vi "TcA01-011_CloneObject.vi"(1 "Input buffer":T3="1", 3 "Invocation info":T2, 5 "error in (no error)":errorcluster, 6 "Add log to result?":bool) -> (16 "Test Data":T1 {"Numeric Measurement" format="%.2f"}, 19 "error out":errorcluster)   [LabVIEW 2009]
doc: "Test case template."
uses:
  Shared/Support_InputBuffer.ctl
  Shared/Support_InvocationInfo.ctl
  Shared/Support_TestData.ctl
  TestClasses/G#SubClass1_class/G#SubClass1.lvclass
  <vilib>/addons/_AddQ/G#Object/G#Object.lvclass
panel:
  in  "Test name":string="TcA01-011 Clone object"
  out "Test result":bool
  out "Result":string
  # "Verify that clone object works."
  # "Sub test case"
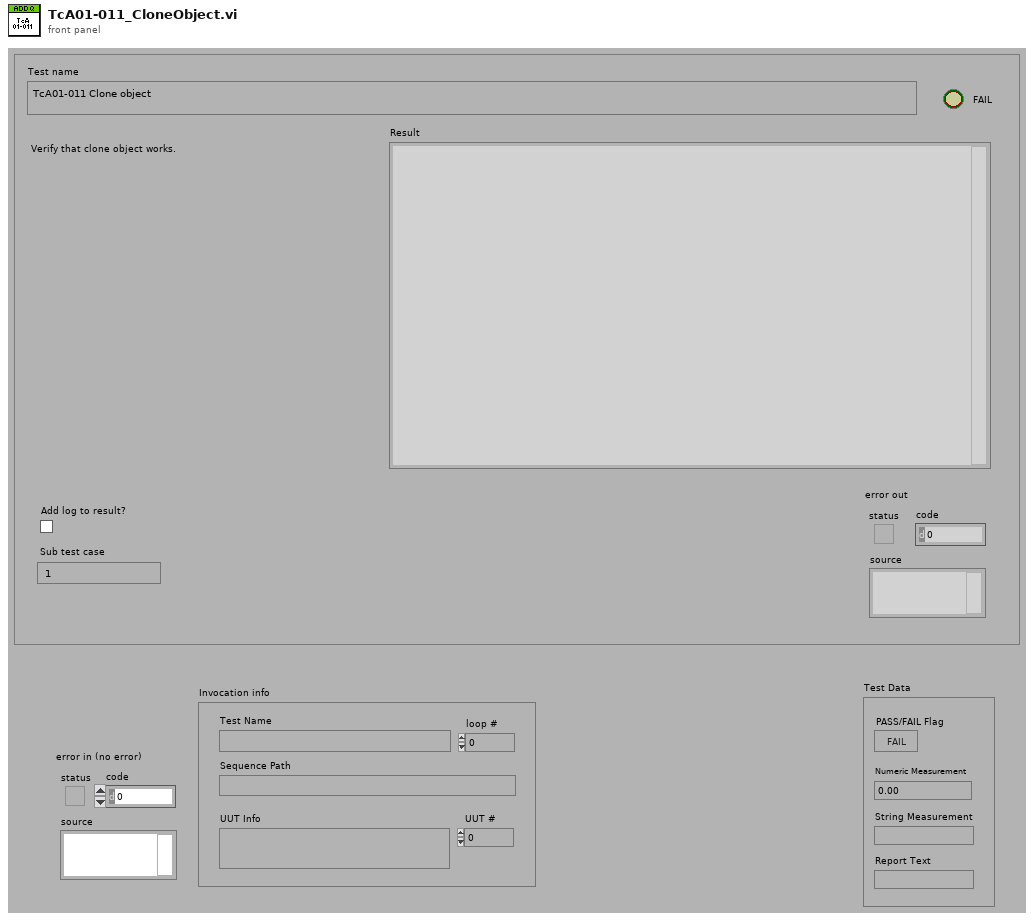
[diagram p1: front panel]
types:
  T1 = typedef "Support_TestData.ctl" = cluster{"PASS/FAIL Flag":bool, "Numeric Measurement":dbl, "String Measurement":string, "Report Text":string}
  T2 = typedef "Support_InvocationInfo.ctl" = cluster{"UUT #":i32, "loop #":i32, "UUT Info":string, "Test Name":string, "Sequence Path":path}
  T3 = typedef "Support_InputBuffer.ctl" = string
  T4 = typedef "Support_ResultType.ctl" = cluster{"Pass":bool, "Comment":string, "MeasurementValue":dbl}
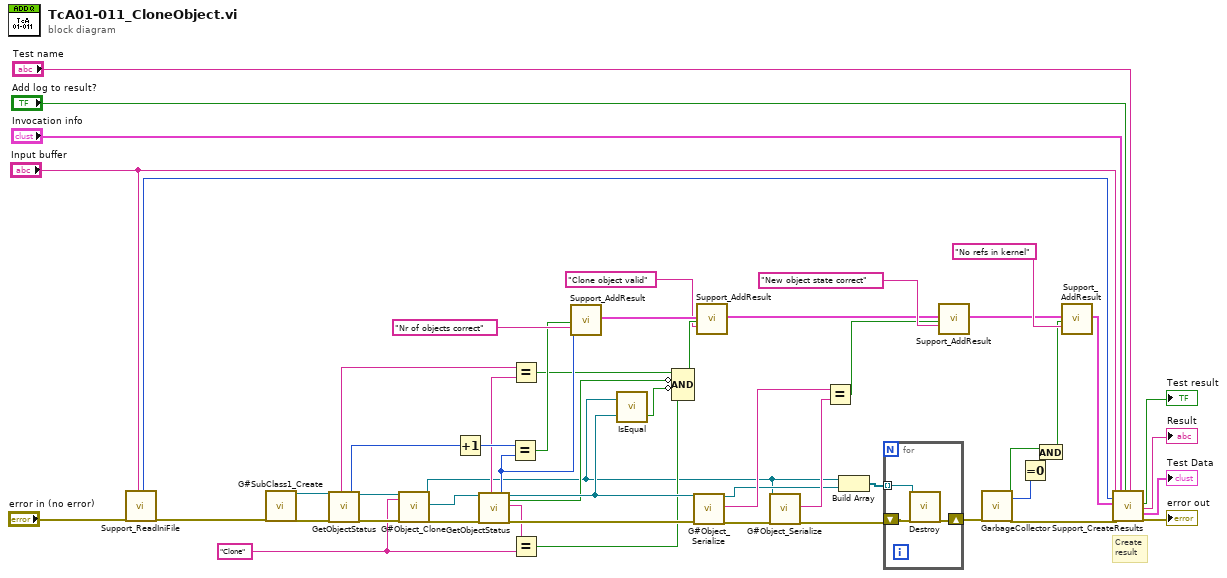
[diagram p0: block diagram]
diagram:
  w1 = "Clone" ("new object name")
  # "Create\nresult"
  n1 = call "Support_ReadIniFile.vi"("error in (no error)"="error in (no error)", "Sub test case"="Input buffer") -> ("Timer start"=w43:u32, "error out"=w34:errorcluster)  [unwired: 10 in, 6 out]
  n2 = call "G#SubClass1_Create.vi"("error in (no error)"=w34) -> ("reference out"=w32:refnum<class "G#SubClass1.lvclass">, "error out"=w33:errorcluster)  [unwired: 16 in, 1 out]
  n3 = call-dynamic "GetObjectStatus.vi"("reference in"=w32, "error in (no error)"=w33) -> ("full class name"=w10:string, "# of objects"=w27:i32, "reference out"=w30:refnum<class "G#SubClass1.lvclass">, "error out"=w31:errorcluster)  [unwired: 6 in, 8 out]
  n4 = call <vilib>:"G#Object_Clone.vi"("reference in"=w30, "new object name"=w1, "error in (no error)"=w31) -> ("reference out"=w3:refnum<class "G#SubClass1.lvclass">, "new object reference out"=w29:refnum<class "G#SubClass1.lvclass">, "error out"=w28:errorcluster)  [unwired: 14 in]
  n5 = Increment(x=w27) -> (x+1=w26:i32)
  n6 = call-dynamic "GetObjectStatus.vi"("reference in"=w29, "error in (no error)"=w28) -> ("full class name"=w11:string, "# of objects"=w25:i32, "reference out"=w19:refnum<class "G#SubClass1.lvclass">, "not a refnum?"=w16:bool, "object name"=w8:string, "error out"=w23:errorcluster)  [unwired: 6 in, 6 out]
  n7 = Equal?(x=w26, y=w25) -> (x = y?=w24:bool)
  n8 = Equal?(x=w10, y=w11) -> (x = y?=w9:bool)
  n9 = Equal?(x=w8, y=w1) -> (x = y?=w7:bool)
  n10 = call "Support_AddResult.vi"("Pass"=w24, "Comment"="Nr of objects correct", "MeasurementValue"=w25) -> ("Results out"=w18:T4[])  [unwired: 16 in]
  n11 = call-dynamic "IsEqual.vi"("is equal to"=w19, "reference in"=w3) -> ("is equal"=w17:bool)  [unwired: 1 out]
  n12 = Compound Arithmetic op=AND(w9, invert w16, invert w17, w7) -> (w15:bool)
  n13 = call-dynamic "G#Object_Serialize.vi"("reference in"=w19, "error in (no error)"=w23) -> ("reference out"=w4:refnum<class "G#SubClass1.lvclass">, "serialized object"=w20:string, "error out"=w22:errorcluster)  [unwired: 14 in, 1 out]
  n14 = call "Support_AddResult.vi"("Results in"=w18, "Pass"=w15, "Comment"="Clone object valid") -> ("Results out"=w13:T4[])  [unwired: 16 in]
  n15 = call-dynamic "G#Object_Serialize.vi"("reference in"=w3, "error in (no error)"=w22) -> ("serialized object"=w21:string, "error out"=w5:errorcluster)  [unwired: 14 in, 2 out]
  n16 = Equal?(x=w20, y=w21) -> (x = y?=w12:bool)
  n17 = Build Array(w3, w4) -> (w2:refnum<class "G#SubClass1.lvclass">[])
  n18 = for {
    shift-right: [w57] -> w6
    shift-left: w5 -> [w56]
    tunnel: w2 -> [w55] mode=indexing
    n19 = call-dynamic "Destroy.vi"("reference in"=w55, "error in (no error)"=w56) -> ("error out"=w57:errorcluster)  [unwired: 16 in, 1 out]
  }
  n20 = call "Support_AddResult.vi"("Results in"=w13, "Pass"=w12, "Comment"="New object state correct") -> ("Results out"=w35:T4[])  [unwired: 16 in]
  n21 = call <vilib>:"GarbageCollector.vi"("error in (no error)"=w6) -> ("OK"=w39:bool, "# of objects killed"=w37:i32, "error out"=w42:errorcluster)  [unwired: 16 in]
  n22 = Equal To 0?(x=w37) -> (x = 0?=w38:bool)
  n23 = And(x=w39, y=w38) -> (x .and. y?=w36:bool)
  n24 = call "Support_AddResult.vi"("Results in"=w35, "Pass"=w36, "Comment"="No refs in kernel") -> ("Results out"=w41:T4[])  [unwired: 16 in]
  n25 = call "Support_CreateResults.vi"("Sub test case"="Input buffer", "Timer start"=w43, "Results"=w41, "error in (no error)"=w42, "Invocation info"="Invocation info", "Add log to result?"="Add log to result?", "Test name"="Test name") -> ("Pass/fail flag"=→"Test result":bool, "Result"=→"Result":string, "Test Data"=→"Test Data":T1, "error out"=→"error out":errorcluster)  [unwired: 9 in]
